vi "Auto Loop 3.vi"(2 "Auto State":u8, 3 "Call Context":T3) -> (0 "Loop 3 Data":T1, 1 "SubState 3":T2)   [LabVIEW 2013]
uses:
  <vilib>/Rock Robotics/WPI/DriverStation/WPI_DriverStationDerivedRobotMode.ctl
  typedefs/subStates.ctl
  typedefs/Loop Datatypes/Loop 3 Datatype.ctl
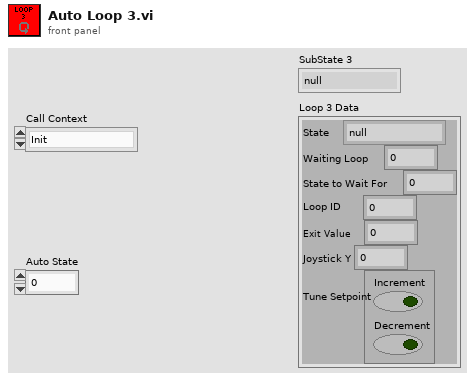
[diagram p1: front panel]
types:
  T1 = typedef "Loop 3 Datatype.ctl" = cluster{"State":T2, "Waiting Loop":i32, "State to Wait For":i32, "Loop ID":i32, "Exit Value":i32, "Joystick Y":dbl, "Tune Setpoint":cluster{"Increment":bool, "Decrement":bool}}
  T2 = typedef "subStates.ctl" = enum16{"null", "wait", "driver control", "auto", "manual override", "hold position", "rotate", "pickup", "pass", "load", "goto shoot", "shoot high goal", "shoot low goal", "cancel arm", "cancel shooter", "end"}
  T3 = typedef "WPI_DriverStationDerivedRobotMode.ctl" = enum16{"Init", "Execute", "Stop"}
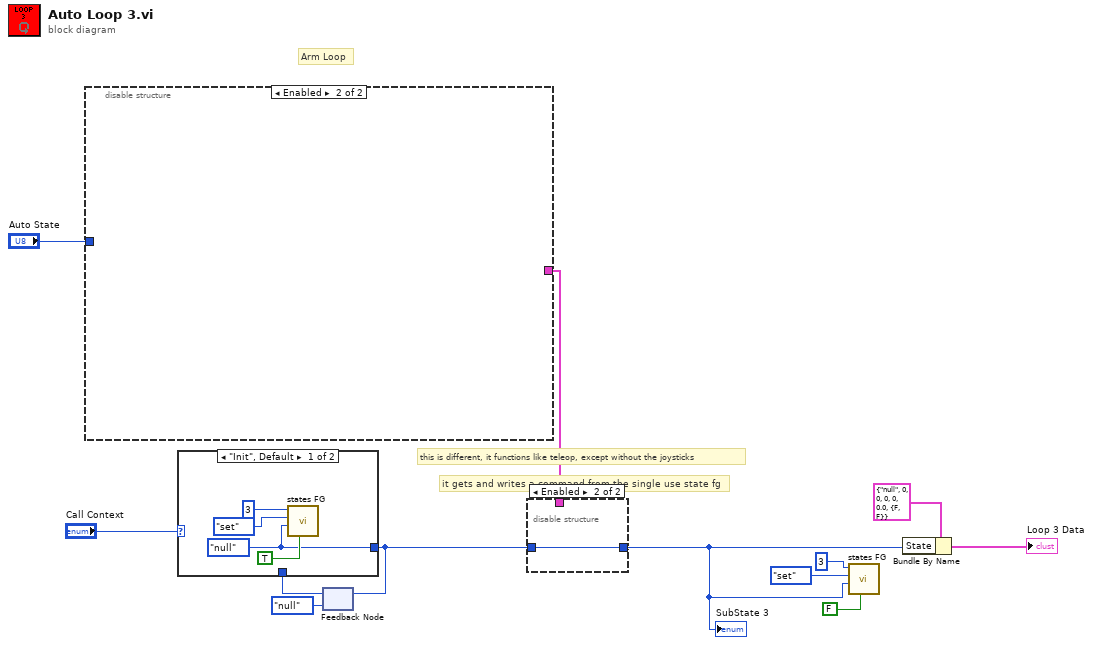
[diagram p0: block diagram]
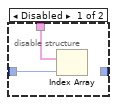
[diagram p2: hidden frame]
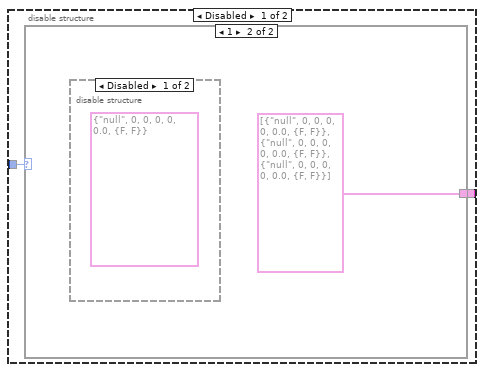
[diagram p3: hidden frame]
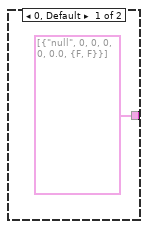
[diagram p4: hidden frame]
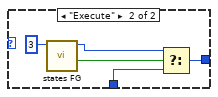
[diagram p6: hidden frame]
diagram:
  # "it gets and writes a command from the single use state fg"
  # "this is different, it functions like teleop, except without the joysticks"
  # "Arm Loop"
  n1 = disable-structure shown="Enabled" {
    disable-tunnel: "Auto State" -> [w14 _]
    disable-tunnel: [w13 _] -> w8
    frame Disabled {
      n2 = case shown="1" w14 {
        tunnel: [T1[] [{"State"=enum."null", "Waiting Loop"=0, "State to Wait For"=0, "Loop ID"=0, "Exit Value"=0, "Joystick Y"=0.0, "Tune Setpoint"={"Increment"=FALSE, "Decrement"=FALSE}}] T1[] [{"State"=enum."null", "Waiting Loop"=0, "State to Wait For"=0, "Loop ID"=0, "Exit Value"=0, "Joystick Y"=0.0, "Tune Setpoint"={"Increment"=FALSE, "Decrement"=FALSE}}, {"State"=enum."null", "Waiting Loop"=0, "State to Wait For"=0, "Loop ID"=0, "Exit Value"=0, "Joystick Y"=0.0, "Tune Setpoint"={"Increment"=FALSE, "Decrement"=FALSE}}, {"State"=enum."null", "Waiting Loop"=0, "State to Wait For"=0, "Loop ID"=0, "Exit Value"=0, "Joystick Y"=0.0, "Tune Setpoint"={"Increment"=FALSE, "Decrement"=FALSE}}]] -> w13
        frame 0, Default {
        }
        frame 1 {
          n3 = disable-structure shown="Disabled" {
            frame Disabled {
              (unwired) T1 {"State"=enum."null", "Waiting Loop"=0, "State to Wait For"=0, "Loop ID"=0, "Exit Value"=0, "Joystick Y"=0.0, "Tune Setpoint"={"Increment"=FALSE, "Decrement"=FALSE}} ("Loop 3 Data")
            }
            frame Enabled {
            }
          }
        }
      }
    }
    frame Enabled {
    }
  }
  n4 = feedback #1(subStates."null" ("subState out")) -> (w10:T2)
  n5 = case shown="\"Init\", Default" "Call Context" {
    tunnel: w10 -> [_ w24]
    tunnel: [w17 w23] -> w9
    frame "Init", Default {
      w17 = subStates."null" ("subState in")
      n6 = call "states FG.vi"("exit in"=TRUE, "subState in"=w17, "menu (get)"=enum16{"set", "get"}."set", "Loop ID"=3) -> ()  [unwired: 4 in, 4 out]
    }
    frame "Execute" {
      n7 = call "states FG.vi"("Loop ID"=3) -> ("exit out"=w22:bool, "subState out"=w21:T2)  [unwired: 7 in, 2 out]
      n8 = Select(t=w21, s=w22, f=w24) -> (s? t:f=w23:T2)
    }
  }
  n9 = feedback-in #1(w9) -> ()
  n10 = disable-structure shown="Enabled" {
    disable-tunnel: w9 -> [w27 w28]
    disable-tunnel: w8 -> [w26 _]
    disable-tunnel: [_ w28] -> w2
    frame Disabled {
      n11 = Index Array(array=w26, index=w27) -> ()  [unwired: 1 out]
    }
    frame Enabled {
    }
  }
  "SubState 3" <- w2
  n12 = call "states FG.vi"("exit in"=FALSE, "subState in"=w2, "menu (get)"=enum16{"set", "get"}."set", "Loop ID"=3) -> ()  [unwired: 4 in, 4 out]
  n13 = Bundle By Name(cluster=T1 {"State"=enum."null", "Waiting Loop"=0, "State to Wait For"=0, "Loop ID"=0, "Exit Value"=0, "Joystick Y"=0.0, "Tune Setpoint"={"Increment"=FALSE, "Decrement"=FALSE}} ("Loop 3 Data"), "State"=w2) -> (→"Loop 3 Data":T1)
